vi "1.vi"() -> ()   [LabVIEW 2017]
uses:
  <vilib>/LabVIEW Interface for Arduino/Type Defs/Pin Mode.ctl
  <vilib>/LabVIEW Interface for Arduino/LabVIEW Interface for Arduino.lvlib
panel:
  in  "stop":bool
  in  "VISA resource":refnum<visa-resource-name>
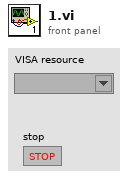
[diagram p1: front panel]
types:
  T1 = typedef "LabVIEW Interface for Arduino.lvlib/Arduino Resource.ctl" = cluster{"VISA resource":refnum<visa-resource-name>, "Board Type":T2, "Connection Type":enum8{"USB / Serial"}, "Bytes Per Packet (15)":u8}
  T2 = typedef "LabVIEW Interface for Arduino.lvlib/Board Type.ctl" = enum16{"Uno", "Dimuelanove w/Atmega 328", "Mega 2560"}
  T3 = typedef "LabVIEW Interface for Arduino.lvlib/Pin Mode.ctl" = enum8{"Input", "Output"}
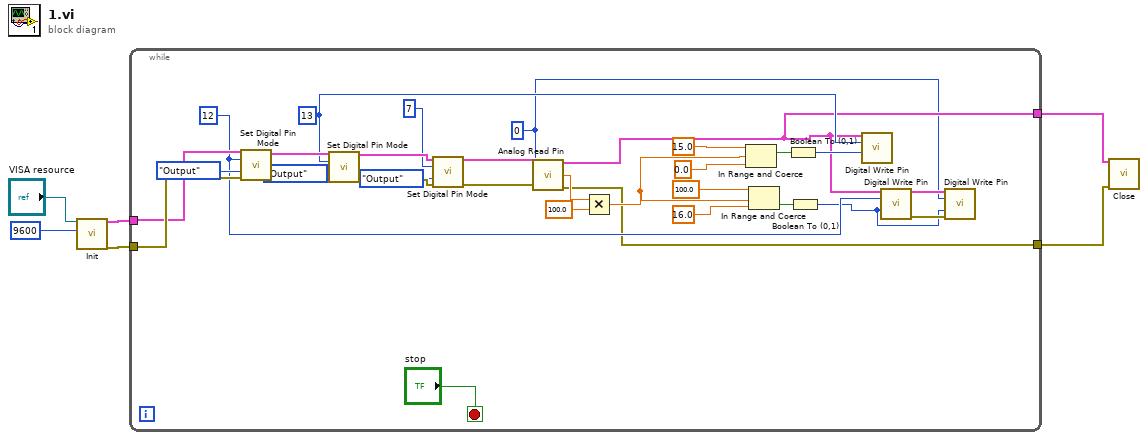
[diagram p0: block diagram]
diagram:
  n1 = call <vilib>:"Init.vi"("VISA resource"="VISA resource", "Baud Rate (115200)"=u32 9600) -> ("Arduino Resource"=w6:T1, "error out"=w5:errorcluster)  [unwired: 16 in]
  n2 = while {
    tunnel: w6 -> [w22]
    tunnel: w5 -> [w36]
    tunnel: [w10] -> w2
    tunnel: [w9] -> w1
    stop <- "stop" stop-if-true
    w7 = u8 0 ("Analog Input Pin (0)")
    w18 = u8 13 ("Digital I/O Pin")
    w17 = u8 12 ("Digital I/O Pin")
    n3 = call <vilib>:"Set Digital Pin Mode.vi"("Arduino Resource"=w22, "Digital I/O Pin"=w17, "Pin Mode (Input)"=Pin_Mode."Output", "error in"=w36) -> ("Arduino Resource"=w37:T1, "error out"=w35:errorcluster)  [unwired: 10 in]
    n4 = call <vilib>:"Set Digital Pin Mode.vi"("Arduino Resource"=w37, "Digital I/O Pin"=w18, "Pin Mode (Input)"=Pin_Mode."Output", "error in"=w35) -> ("Arduino Resource"=w25:T1, "error out"=w24:errorcluster)  [unwired: 10 in]
    n5 = call <vilib>:"Set Digital Pin Mode.vi"("Arduino Resource"=w25, "Digital I/O Pin"=u8 7, "Pin Mode (Input)"=Pin_Mode."Output", "error in"=w24) -> ("Arduino Resource"=w21:T1, "error out"=w20:errorcluster)  [unwired: 10 in]
    n6 = call <vilib>:"Analog Read Pin.vi"("Arduino Resource"=w21, "Analog Input Pin (0)"=w7, "error in"=w20) -> ("Arduino Resource"=w10:T1, "Voltage"=w16:dbl, "error out"=w9:errorcluster)  [unwired: 10 in]
    n7 = Multiply(x=w16, y=100.0) -> (x*y=w14:dbl)
    n8 = In Range and Coerce(upper limit=15.0, x=w14, lower limit=0.0) -> (In Range?=w28:bool)  [unwired: 1 out]
    n9 = In Range and Coerce(upper limit=100.0, x=w14, lower limit=16.0) -> (In Range?=w27:bool)  [unwired: 1 out]
    n10 = Boolean To (0,1)(Boolean=w28) -> (0, 1=w26:i16)
    n11 = Boolean To (0,1)(Boolean=w27) -> (0, 1=w8:i16)
    n12 = call <vilib>:"Digital Write Pin.vi"("Arduino Resource"=w10, "Digital I/O Pin (0)"=w18, "Value (0)"=w26) -> ()  [unwired: 11 in, 2 out]
    n13 = call <vilib>:"Digital Write Pin.vi"("Arduino Resource"=w10, "Digital I/O Pin (0)"=w17, "Value (0)"=w8) -> ("Arduino Resource"=w13:T1, "error out"=w12:errorcluster)  [unwired: 11 in]
    n14 = call <vilib>:"Digital Write Pin.vi"("Arduino Resource"=w13, "Digital I/O Pin (0)"=w7, "Value (0)"=w8, "error in"=w12) -> ()  [unwired: 10 in, 2 out]
  }
  n15 = call <vilib>:"Close.vi"("Arduino Resource"=w2, "error in"=w1) -> ()  [unwired: 13 in, 1 out]
